vi "Get Broken VIs.vi"(8 "error in (no error)":errorcluster, 11 "SDIST in":refnum<class "NI_AB_API_SDIST.lvclass">) -> (0 "error out":errorcluster, 1 "before build?":bool, 2 "Broken VI List":string[](array[string]), 3 "SDIST out":refnum<class "NI_AB_API_SDIST.lvclass">, 5 "Has errors?":bool=TRUE)   [LabVIEW 2020, in "NI_AB_API_SDIST.lvclass"]
uses:
  <vilib>/AppBuilder/AB_API/SDIST/NI_AB_API_SDIST.lvclass
  <vilib>/AppBuilder/AB_API/Build/NI_AB_API_Build.lvclass
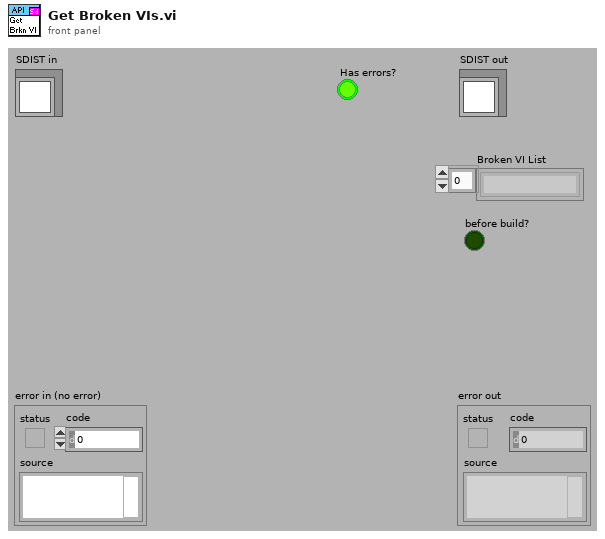
[diagram p1: front panel]
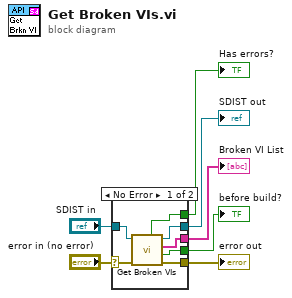
[diagram p0: block diagram]
diagram:
  n1 = case shown="No Error" "error in (no error)" {
    selector: "error in (no error)" -> [w8 w16]
    tunnel: [w9 w16] -> w6
    tunnel: [w13 w15] -> w4
    tunnel: "SDIST in" -> [w14 w15]
    tunnel: [w12 _] -> w3
    tunnel: [w11 _] -> w2
    tunnel: [w10 _] -> w1
    frame No Error {
      n2 = call-parent "Get Broken VIs.vi"("error in (no error)"=w8, "NI_AB_API_Build in"=w14) -> ("error out"=w9:errorcluster, "before build?"=w10:bool, "Broken VI List"=w11:string[], "NI_AB_API_Build out"=w13:refnum<class "NI_AB_API_SDIST.lvclass">, "Has errors?"=w12:bool)  [unwired: 5 in]
    }
    frame Error {
    }
  }
  "error out" <- w6
  "SDIST out" <- w4
  "Has errors?" <- w3
  "Broken VI List" <- w2
  "before build?" <- w1
